vi "Sort Transactions By Source.vi"(10 "Transactions In":T2[](array[typedef])=[{"Dataset Source"=enum."LBCB 1", "Dataset Type"=enum."Displacement", "Hold"=TRUE, "Volts"=FALSE, "Tag"=""}, {"Dataset Source"=enum."LBCB 1", "Dataset Type"=enum."Force", "Hold"=TRUE, "Volts"=FALSE, "Tag"=""}, {"Dataset Source"=enum."LBCB 1", "Dataset Type"=enum."LVDT", "Hold"=TRUE, "Volts"=FALSE, "Tag"=""}, {"Dataset Source"=enum."LBCB 1", "Dataset Type"=enum."Load Cell", "Hold"=TRUE, "Volts"=FALSE, "Tag"=""}, {"Dataset Source"=enum."LBCB 2", "Dataset Type"=enum."Displacement", "Hold"=TRUE, "Volts"=FALSE, "Tag"=""}, {"Dataset Source"=enum."LBCB 2", "Dataset Type"=enum."Force", "Hold"=TRUE, "Volts"=FALSE, "Tag"=""}, {"Dataset Source"=enum."LBCB 2", "Dataset Type"=enum."LVDT", "Hold"=TRUE, "Volts"=FALSE, "Tag"=""}, {"Dataset Source"=enum."LBCB 2", "Dataset Type"=enum."Load Cell", "Hold"=TRUE, "Volts"=FALSE, "Tag"=""}, {"Dataset Source"=enum."Combined", "Dataset Type"=enum."Displacement", "Hold"=TRUE, "Volts"=FALSE, "Tag"=""}, {"Dataset Source"=enum."Combined", "Dataset Type"=enum."Force", "Hold"=TRUE, "Volts"=FALSE, "Tag"=""}, {"Dataset Source"=enum."LBCB 1", "Dataset Type"=enum."Actuator Command", "Hold"=FALSE, "Volts"=FALSE, "Tag"=""}, {"Dataset Source"=enum."LBCB 1", "Dataset Type"=enum."Displacement Command", "Hold"=FALSE, "Volts"=FALSE, "Tag"=""}, {"Dataset Source"=enum."LBCB 2", "Dataset Type"=enum."Actuator Command", "Hold"=FALSE, "Volts"=FALSE, "Tag"=""}, {"Dataset Source"=enum."LBCB 2", "Dataset Type"=enum."Displacement Command", "Hold"=FALSE, "Volts"=FALSE, "Tag"=""}, {"Dataset Source"=enum."Combined", "Dataset Type"=enum."Displacement Command", "Hold"=FALSE, "Volts"=FALSE, "Tag"=""}]) -> (2 "Transactions Out":T2[](array[typedef])=[{"Dataset Source"=enum."LBCB 1", "Dataset Type"=enum."Displacement", "Hold"=TRUE, "Volts"=FALSE, "Tag"=""}, {"Dataset Source"=enum."LBCB 1", "Dataset Type"=enum."Force", "Hold"=TRUE, "Volts"=FALSE, "Tag"=""}, {"Dataset Source"=enum."LBCB 1", "Dataset Type"=enum."LVDT", "Hold"=TRUE, "Volts"=FALSE, "Tag"=""}, {"Dataset Source"=enum."LBCB 1", "Dataset Type"=enum."Load Cell", "Hold"=TRUE, "Volts"=FALSE, "Tag"=""}, {"Dataset Source"=enum."LBCB 2", "Dataset Type"=enum."Displacement", "Hold"=TRUE, "Volts"=FALSE, "Tag"=""}, {"Dataset Source"=enum."LBCB 2", "Dataset Type"=enum."Force", "Hold"=TRUE, "Volts"=FALSE, "Tag"=""}, {"Dataset Source"=enum."LBCB 2", "Dataset Type"=enum."LVDT", "Hold"=TRUE, "Volts"=FALSE, "Tag"=""}, {"Dataset Source"=enum."LBCB 2", "Dataset Type"=enum."Load Cell", "Hold"=TRUE, "Volts"=FALSE, "Tag"=""}, {"Dataset Source"=enum."Combined", "Dataset Type"=enum."Displacement", "Hold"=TRUE, "Volts"=FALSE, "Tag"=""}, {"Dataset Source"=enum."Combined", "Dataset Type"=enum."Force", "Hold"=TRUE, "Volts"=FALSE, "Tag"=""}, {"Dataset Source"=enum."LBCB 1", "Dataset Type"=enum."Actuator Command", "Hold"=FALSE, "Volts"=FALSE, "Tag"=""}, {"Dataset Source"=enum."LBCB 1", "Dataset Type"=enum."Displacement Command", "Hold"=FALSE, "Volts"=FALSE, "Tag"=""}, {"Dataset Source"=enum."LBCB 2", "Dataset Type"=enum."Actuator Command", "Hold"=FALSE, "Volts"=FALSE, "Tag"=""}, {"Dataset Source"=enum."LBCB 2", "Dataset Type"=enum."Displacement Command", "Hold"=FALSE, "Volts"=FALSE, "Tag"=""}, {"Dataset Source"=enum."Combined", "Dataset Type"=enum."Displacement Command", "Hold"=FALSE, "Volts"=FALSE, "Tag"=""}, {"Dataset Source"=enum."LBCB 1", "Dataset Type"=enum."Displacement", "Hold"=TRUE, "Volts"=FALSE, "Tag"=""}, {"Dataset Source"=enum."LBCB 1", "Dataset Type"=enum."Force", "Hold"=TRUE, "Volts"=FALSE, "Tag"=""}, {"Dataset Source"=enum."LBCB 1", "Dataset Type"=enum."LVDT", "Hold"=TRUE, "Volts"=FALSE, "Tag"=""}, {"Dataset Source"=enum."LBCB 1", "Dataset Type"=enum."Load Cell", "Hold"=TRUE, "Volts"=FALSE, "Tag"=""}, {"Dataset Source"=enum."LBCB 1", "Dataset Type"=enum."Actuator Command", "Hold"=FALSE, "Volts"=FALSE, "Tag"=""}, {"Dataset Source"=enum."LBCB 1", "Dataset Type"=enum."Displacement Command", "Hold"=FALSE, "Volts"=FALSE, "Tag"=""}, {"Dataset Source"=enum."LBCB 1", "Dataset Type"=enum."Displacement", "Hold"=TRUE, "Volts"=FALSE, "Tag"=""}, {"Dataset Source"=enum."LBCB 1", "Dataset Type"=enum."Force", "Hold"=TRUE, "Volts"=FALSE, "Tag"=""}, {"Dataset Source"=enum."LBCB 1", "Dataset Type"=enum."LVDT", "Hold"=TRUE, "Volts"=FALSE, "Tag"=""}, {"Dataset Source"=enum."LBCB 1", "Dataset Type"=enum."Load Cell", "Hold"=TRUE, "Volts"=FALSE, "Tag"=""}, {"Dataset Source"=enum."LBCB 2", "Dataset Type"=enum."Displacement", "Hold"=TRUE, "Volts"=FALSE, "Tag"=""}, {"Dataset Source"=enum."LBCB 2", "Dataset Type"=enum."Force", "Hold"=TRUE, "Volts"=FALSE, "Tag"=""}, {"Dataset Source"=enum."LBCB 2", "Dataset Type"=enum."LVDT", "Hold"=TRUE, "Volts"=FALSE, "Tag"=""}, {"Dataset Source"=enum."LBCB 2", "Dataset Type"=enum."Load Cell", "Hold"=TRUE, "Volts"=FALSE, "Tag"=""}, {"Dataset Source"=enum."Combined", "Dataset Type"=enum."Displacement", "Hold"=TRUE, "Volts"=FALSE, "Tag"=""}, {"Dataset Source"=enum."Combined", "Dataset Type"=enum."Force", "Hold"=TRUE, "Volts"=FALSE, "Tag"=""}, {"Dataset Source"=enum."LBCB 1", "Dataset Type"=enum."Actuator Command", "Hold"=FALSE, "Volts"=FALSE, "Tag"=""}, {"Dataset Source"=enum."LBCB 1", "Dataset Type"=enum."Displacement Command", "Hold"=FALSE, "Volts"=FALSE, "Tag"=""}, {"Dataset Source"=enum."LBCB 2", "Dataset Type"=enum."Actuator Command", "Hold"=FALSE, "Volts"=FALSE, "Tag"=""}, {"Dataset Source"=enum."LBCB 2", "Dataset Type"=enum."Displacement Command", "Hold"=FALSE, "Volts"=FALSE, "Tag"=""}, {"Dataset Source"=enum."Combined", "Dataset Type"=enum."Displacement Command", "Hold"=FALSE, "Volts"=FALSE, "Tag"=""}, {"Dataset Source"=enum."LBCB 2", "Dataset Type"=enum."Displacement", "Hold"=TRUE, "Volts"=FALSE, "Tag"=""}, {"Dataset Source"=enum."LBCB 2", "Dataset Type"=enum."Force", "Hold"=TRUE, "Volts"=FALSE, "Tag"=""}, {"Dataset Source"=enum."LBCB 2", "Dataset Type"=enum."LVDT", "Hold"=TRUE, "Volts"=FALSE, "Tag"=""}, {"Dataset Source"=enum."LBCB 2", "Dataset Type"=enum."Load Cell", "Hold"=TRUE, "Volts"=FALSE, "Tag"=""}, {"Dataset Source"=enum."LBCB 2", "Dataset Type"=enum."Actuator Command", "Hold"=FALSE, "Volts"=FALSE, "Tag"=""}, {"Dataset Source"=enum."LBCB 2", "Dataset Type"=enum."Displacement Command", "Hold"=FALSE, "Volts"=FALSE, "Tag"=""}, {"Dataset Source"=enum."LBCB 1", "Dataset Type"=enum."Displacement", "Hold"=TRUE, "Volts"=FALSE, "Tag"=""}, {"Dataset Source"=enum."LBCB 1", "Dataset Type"=enum."Force", "Hold"=TRUE, "Volts"=FALSE, "Tag"=""}, {"Dataset Source"=enum."LBCB 1", "Dataset Type"=enum."LVDT", "Hold"=TRUE, "Volts"=FALSE, "Tag"=""}, {"Dataset Source"=enum."LBCB 1", "Dataset Type"=enum."Load Cell", "Hold"=TRUE, "Volts"=FALSE, "Tag"=""}, {"Dataset Source"=enum."LBCB 2", "Dataset Type"=enum."Displacement", "Hold"=TRUE, "Volts"=FALSE, "Tag"=""}, {"Dataset Source"=enum."LBCB 2", "Dataset Type"=enum."Force", "Hold"=TRUE, "Volts"=FALSE, "Tag"=""}, {"Dataset Source"=enum."LBCB 2", "Dataset Type"=enum."LVDT", "Hold"=TRUE, "Volts"=FALSE, "Tag"=""}, {"Dataset Source"=enum."LBCB 2", "Dataset Type"=enum."Load Cell", "Hold"=TRUE, "Volts"=FALSE, "Tag"=""}, {"Dataset Source"=enum."Combined", "Dataset Type"=enum."Displacement", "Hold"=TRUE, "Volts"=FALSE, "Tag"=""}, {"Dataset Source"=enum."Combined", "Dataset Type"=enum."Force", "Hold"=TRUE, "Volts"=FALSE, "Tag"=""}, {"Dataset Source"=enum."LBCB 1", "Dataset Type"=enum."Actuator Command", "Hold"=FALSE, "Volts"=FALSE, "Tag"=""}, {"Dataset Source"=enum."LBCB 1", "Dataset Type"=enum."Displacement Command", "Hold"=FALSE, "Volts"=FALSE, "Tag"=""}, {"Dataset Source"=enum."LBCB 2", "Dataset Type"=enum."Actuator Command", "Hold"=FALSE, "Volts"=FALSE, "Tag"=""}, {"Dataset Source"=enum."LBCB 2", "Dataset Type"=enum."Displacement Command", "Hold"=FALSE, "Volts"=FALSE, "Tag"=""}, {"Dataset Source"=enum."Combined", "Dataset Type"=enum."Displacement Command", "Hold"=FALSE, "Volts"=FALSE, "Tag"=""}, {"Dataset Source"=enum."Combined", "Dataset Type"=enum."Displacement", "Hold"=TRUE, "Volts"=FALSE, "Tag"=""}, {"Dataset Source"=enum."Combined", "Dataset Type"=enum."Force", "Hold"=TRUE, "Volts"=FALSE, "Tag"=""}, {"Dataset Source"=enum."Combined", "Dataset Type"=enum."Displacement Command", "Hold"=FALSE, "Volts"=FALSE, "Tag"=""}, {"Dataset Source"=enum."LBCB 1", "Dataset Type"=enum."Displacement", "Hold"=TRUE, "Volts"=FALSE, "Tag"=""}, {"Dataset Source"=enum."LBCB 1", "Dataset Type"=enum."Force", "Hold"=TRUE, "Volts"=FALSE, "Tag"=""}, {"Dataset Source"=enum."LBCB 1", "Dataset Type"=enum."LVDT", "Hold"=TRUE, "Volts"=FALSE, "Tag"=""}, {"Dataset Source"=enum."LBCB 1", "Dataset Type"=enum."Load Cell", "Hold"=TRUE, "Volts"=FALSE, "Tag"=""}, {"Dataset Source"=enum."LBCB 2", "Dataset Type"=enum."Displacement", "Hold"=TRUE, "Volts"=FALSE, "Tag"=""}, {"Dataset Source"=enum."LBCB 2", "Dataset Type"=enum."Force", "Hold"=TRUE, "Volts"=FALSE, "Tag"=""}, {"Dataset Source"=enum."LBCB 2", "Dataset Type"=enum."LVDT", "Hold"=TRUE, "Volts"=FALSE, "Tag"=""}, {"Dataset Source"=enum."LBCB 2", "Dataset Type"=enum."Load Cell", "Hold"=TRUE, "Volts"=FALSE, "Tag"=""}, {"Dataset Source"=enum."Combined", "Dataset Type"=enum."Displacement", "Hold"=TRUE, "Volts"=FALSE, "Tag"=""}, {"Dataset Source"=enum."Combined", "Dataset Type"=enum."Force", "Hold"=TRUE, "Volts"=FALSE, "Tag"=""}, {"Dataset Source"=enum."LBCB 1", "Dataset Type"=enum."Actuator Command", "Hold"=FALSE, "Volts"=FALSE, "Tag"=""}, {"Dataset Source"=enum."LBCB 1", "Dataset Type"=enum."Displacement Command", "Hold"=FALSE, "Volts"=FALSE, "Tag"=""}, {"Dataset Source"=enum."LBCB 2", "Dataset Type"=enum."Actuator Command", "Hold"=FALSE, "Volts"=FALSE, "Tag"=""}, {"Dataset Source"=enum."LBCB 2", "Dataset Type"=enum."Displacement Command", "Hold"=FALSE, "Volts"=FALSE, "Tag"=""}, {"Dataset Source"=enum."Combined", "Dataset Type"=enum."Displacement Command", "Hold"=FALSE, "Volts"=FALSE, "Tag"=""}])   [LabVIEW 2013]
uses:
  Dataset Transaction Id.ctl
  Dataset Source.ctl
  Dataset Type.ctl
  Apps/Yes No Button.ctl
panel:
  in  "Sorted Source":T1[](array[typedef])=[enum."Combined", enum."LBCB 1", enum."LBCB 2", enum."External Sensors"]
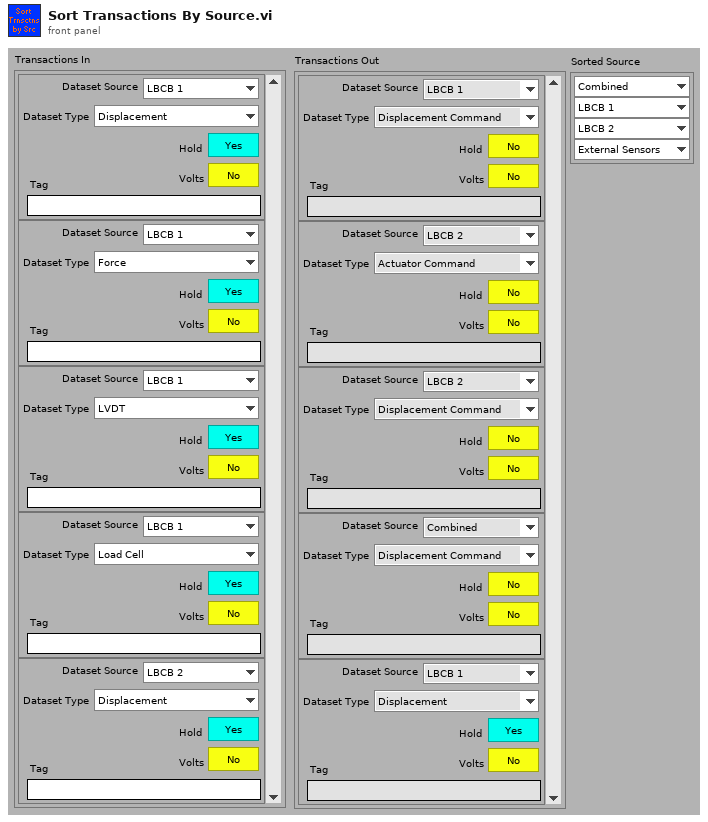
[diagram p1: front panel]
types:
  T1 = typedef "Dataset Source.ctl" = enum16{"LBCB 1", "LBCB 2", "Combined", "External Sensors"}
  T2 = typedef "Dataset Transaction Id.ctl" = cluster{"Dataset Source":T1, "Dataset Type":T3, "Hold":T4, "Volts":T4, "Tag":string}
  T3 = typedef "Dataset Type.ctl" = enum16{"LVDT", "Load Cell", "Actuator Command", "Servo Error", "Displacement Command", "Displacement", "Force"}
  T4 = typedef "Yes No Button.ctl" = bool
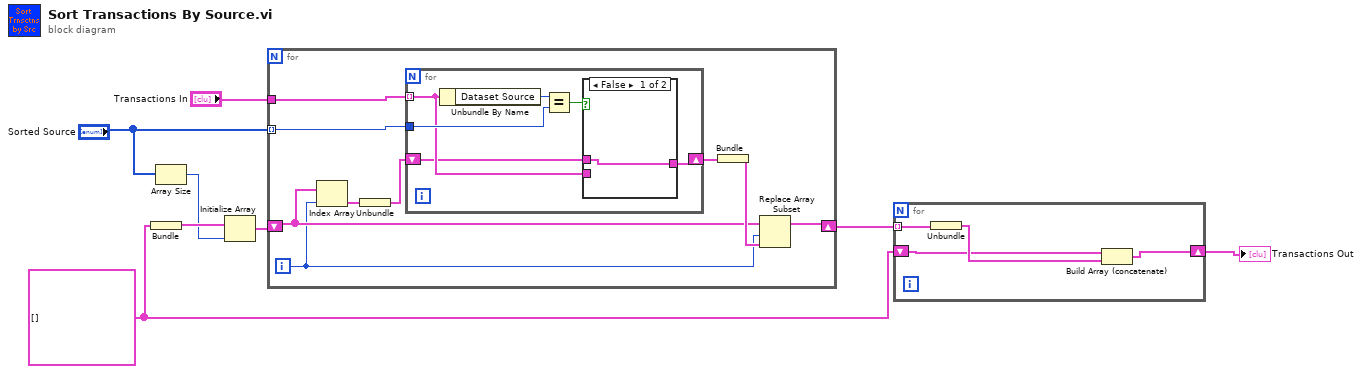
[diagram p0: block diagram]
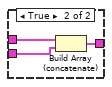
[diagram p2: hidden frame]
diagram:
  w1 = T2[] []
  n1 = Bundle(w1) -> (w8:cluster{T2[]})  [unwired: 1 in]
  n2 = Array Size(array="Sorted Source") -> (size(s)=w7:i32)
  n3 = Initialize Array(w8, w7) -> (w6:cluster{T2[]}[])
  n4 = for {
    shift-right: [w13] -> w3
    shift-left: w6 -> [w12]
    tunnel: "Sorted Source" -> [w17] mode=indexing
    tunnel: "Transactions In" -> [w16]
    i -> [w11]
    n5 = Index Array(array=w12, index=w11) -> (element=w10:cluster{T2[]})
    n6 = Unbundle(w10) -> (w9:T2[])
    n7 = for {
      tunnel: w17 -> [w22]
      tunnel: w16 -> [w19] mode=indexing
      shift-right: [w20] -> w14
      shift-left: w9 -> [w18]
      n8 = Unbundle By Name(w19) -> ("Dataset Source"=w23:T1)
      n9 = Equal?(x=w23, y=w22) -> (x = y?=w21:bool)
      n10 = case shown="False" w21 {
        tunnel: [w24 w27] -> w20
        tunnel: w19 -> [_ w26]
        tunnel: w18 -> [w24 w25]
        frame False {
        }
        frame True {
          n11 = Build Array (concatenate)(w25, w26) -> (w27:T2[])
        }
      }
    }
    n12 = Bundle(w14) -> (w15:cluster{T2[]})  [unwired: 1 in]
    n13 = Replace Array Subset(array=w12, new element=w15, index=w11) -> (w13:cluster{T2[]}[])
  }
  n14 = for {
    tunnel: w3 -> [w31] mode=indexing
    shift-right: [w29] -> w2
    shift-left: w1 -> [w28]
    n15 = Unbundle(w31) -> (w30:T2[])
    n16 = Build Array (concatenate)(w28, w30) -> (w29:T2[])
  }
  "Transactions Out" <- w2
